vi "SiosIfmCancelBlock.vi"(1 "Device Number":i32) -> (0 "Success":i32)   [LabVIEW 2009]
uses:
  siosifm.dll
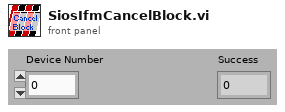
[diagram p1: front panel]
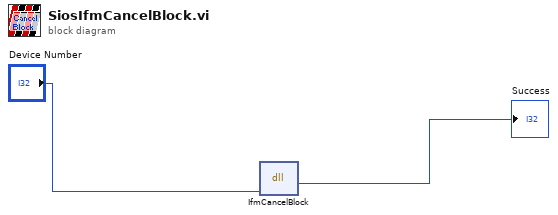
[diagram p0: block diagram]
diagram:
  n1 = dll-call lib="C:/WORK/Artem/RE-10/SIOS_IfmDLL/siosifm.dll" fn="IfmCancelBlock"("devNumber"="Device Number") -> ("Success"=→"Success":i32)  [unwired: 4 in, 2 out]
